vi "PH_PSDBController.Set PSDB Error.vi"(0 "i ref in":refnum<vi>, 2 "Data Status":T1 items=["no info", "no Data collection", "no problem", "Error getting the ID", "Error writing Data", "Error getting the subsystem", "Error getting the Shot ID", "Error getting the Shot Types", "Error getting the Experiments", "Error verifying wanted Shottype", "Error verifying wanted Experiment"], 5 "error in":errorcluster) -> (14 "i ref out":refnum<vi>, 19 "error out":errorcluster)   [LabVIEW 2014, in "PH_PSDBController.lvlib"]
doc: "This VI sets the Error to own attributes and the GUI. Handle with care: It is using the semaphores writing the data to own attributes."
uses:
  PH_PSDBController.lvlib
  PH_PSDBWriter/PH_PSDBWriter.Data Status.ctl
  PH_PSDBWriter/PH_PSDBWriter.lvlib
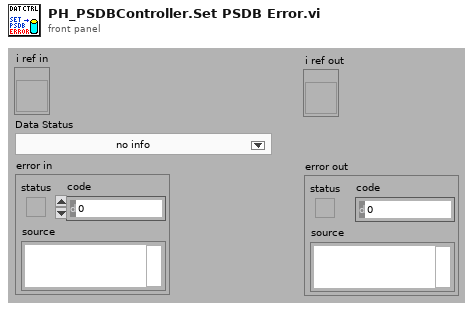
[diagram p1: front panel]
types:
  T1 = typedef "PH_PSDBWriter.lvlib/PH_PSDBWriter.Data Status.ctl" = i16
  T2 = typedef "PH_PSDBController.lvlib/PH_PSDBController.i attribute.ctl" = cluster{"GUI Refs":cluster{"Data Status":refnum<vi>, "Current Shot ID":refnum<vi>, "active Subsystems":refnum<vi>, "Experiment Description":refnum<vi>, "Shot Comment":refnum<vi>, "Experiment":refnum<vi>, "Shottype":refnum<vi>, "Sequencer SM State":refnum<vi>, "Instances with Errors":refnum<vi>}, "Service ID Shot ID":i32, "Service ID wanted Subsystem":i32, "Data Status":T1, "Shotinformation":cluster{"Current Experiment ID":i32, "Current Shot Type":i32, "Current Comment":string}, "Data taking?":bool, "Service ID current Shottype":i32, "Service ID current Experiment":i32, "Service ID currentShot Comment":i32, "Service ID possible Shottypes":i32, "Service ID possible Experiments":i32, "possible Experiments":T3[], "possible Shottypes":T3[], "List":cluster{"Info":cluster{"Instance":string, "Data Status":T1}[], "GUI Ref":refnum<vi>, "Classname":string}[], "Subsystems Off?":cluster{"PHELIX_Beamline_fs_YLF_BL_Status":bool, "PHELIX_Beamline_ns_BL_Status":bool, "PHELIX_Beamline_PA_Input_BL_Status":bool, "PHELIX_Beamline_PA_MA_BL_Status":bool, "PHELIX_Beamline_MA_Z6_BL_Status":bool, "PHELIX_Beamline_MA_LB_BL_Status":bool, "PHELIX_Beamline_PA_LL_BL_Status":bool}, "PSDB Credentials":T4}
  T3 = typedef "PSDB.lvlib/PSDB_Info.ctl" = cluster{"Name":string, "Description":string, "ID":i32}
  T4 = typedef "PH_Common.lvlib/PH_Connection.PSDB Credentials.ctl" = cluster{"PW":string, "ID":string, "DS":string}
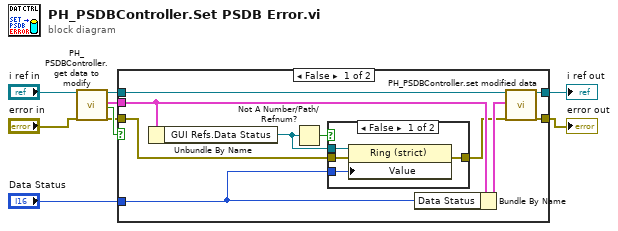
[diagram p0: block diagram]
diagram:
  n1 = call "PH_PSDBController.get data to modify.vi"("i ref in"="i ref in", "error in (no error)"="error in") -> ("i ref out"=w2:refnum<vi>, "i attribute"=w9:T2, "timed out"=w8:bool, "error out"=w5:errorcluster)  [unwired: 14 in]
  n2 = case shown="False" w8 {
    tunnel: w2 -> [w19 w26]
    tunnel: [w18 w26] -> w4
    tunnel: w5 -> [w13 w25]
    tunnel: [w17 w25] -> w7
    tunnel: w9 -> [w15 _]
    tunnel: "Data Status" -> [w14 _]
    frame False {
      n3 = Unbundle By Name(w15) -> ("GUI Refs.Data Status"=w10:refnum<vi>)
      n4 = Not A Number/Path/Refnum?(number/path/refnum=w10) -> (NaN/Path/Refnum?=w11:bool)
      n5 = case shown="False" w11 {
        tunnel: w10 -> [w23 _]
        tunnel: w14 -> [w22 _]
        tunnel: w13 -> [w21 w24]
        tunnel: [w20 w24] -> w12
        frame False {
          n6 = property class="Ring (strict)"(reference=w23, error in=w21, "Value"=w22) -> (error out=w20:errorcluster)  [unwired: 1 out]
        }
        frame True {
        }
      }
      n7 = Bundle By Name(cluster=w15, "Data Status"=w14) -> (w16:T2)
      n8 = call "PH_PSDBController.set modified data.vi"("i ref in"=w19, "i attribute"=w16, "error in (no error)"=w12) -> ("i ref out"=w18:refnum<vi>, "error out"=w17:errorcluster)  [unwired: 15 in]
    }
    frame True {
    }
  }
  "error out" <- w7
  "i ref out" <- w4
